vi "Main.vi"(11 "Module Admin":refnum<class "Delacor_lib_QMH_Module Admin.lvclass">) -> ()   [LabVIEW 2020, in "Config.lvlib"]
doc: "This template is based off of the Queued Message Handler design pattern and the Queued Message Handler project template that ships with LabVIEW.\n\nThe main difference is that the queue is private to this module and communication between modules is performed via Broadcast and Request events.\n\nRequest events are wrapped in public API methods and are handled in the Event Handling Loop (EHL) of this VI. Any module can register for Broadcast events sent by this module. The EHL generates messages based on user interface actions.\n\nThe Message Handling Loop (MHL) processes messages generated by the EHL, or by other messages. The messages are string values, so new messages can be added easily to the Message Cases case structure in the MHL. Each message cluster can also provide an optional value for Message Data, which is a variant that can be converted to whatever message-specific data is required.\n_____\nBased on Delacor QMH Project Template 5.0.0.82."
uses:
  Config.lvlib
  <vilib>/Delacor/Delacor QMH/Libraries/Module Admin_class/Delacor_lib_QMH_Module Admin.lvclass
  Acquisition/SignalConfig--cluster.ctl
  Module Data--cluster.ctl
  Stop Argument--cluster.ctl
  <vilib>/Delacor/Delacor QMH/Libraries/Message Queue_class/Delacor_lib_QMH_Message Queue.lvclass/Delacor_lib_QMH_Message Queue.ctl
  <vilib>/Delacor/Delacor QMH/Libraries/Module Admin_class/Delacor_lib_QMH_Module Admin.lvclass/Delacor_lib_QMH_Module Admin.ctl
  Save Config Argument--cluster.ctl
  Cancel config Argument--cluster.ctl
  Load Config Argument--cluster.ctl
  Load Config (Reply Payload)--cluster.ctl
  Config Loaded from DB Argument--cluster.ctl
  <vilib>/Utility/miscctls.llb/LVPointTypeDef.ctl
  <vilib>/Delacor/Delacor QMH/Libraries/Message Queue_class/Delacor_lib_QMH_Enqueue Message (Single).vi
  <vilib>/Delacor/Delacor QMH/Libraries/Module Admin_class/Delacor_lib_QMH_Get External Launch.vi
  <vilib>/Utility/error.llb/Error Cluster From Error Code.vi
  <vilib>/ErrorRing/Error Ring.xnode
  <vilib>/Delacor/Delacor QMH/Libraries/Message Queue_class/Delacor_lib_QMH_Message Queue.lvclass
  DataBase/DataBase.lvlib
panel:
  in  "SignalConfig":T1={"VPP"=0, "Frecuency"=50.0, "Offset"=0.0, "signal type"=enum."Sine Wave"}
  in  "Save":bool
  in  "Cancel":bool
  out "error out":errorcluster
  out "Status":string
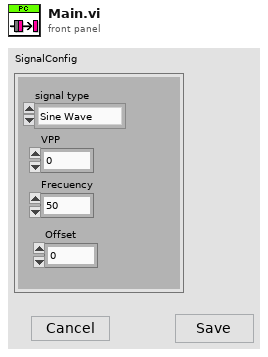
[diagram p1: front panel]
types:
  T1 = typedef "SignalConfig--cluster.ctl" = cluster{"VPP":i32, "Frecuency":dbl, "Offset":dbl, "signal type":enum16{"Sine Wave", "Triangle Wave", "Square Wave", "Sawtooth Wave"}}
  T2 = typedef "Config.lvlib/Request Events--cluster.ctl" = cluster{"Stop Module":refnum<user-event>, "Show Panel":refnum<user-event>, "Hide Panel":refnum<user-event>, "Get Module Execution Status":refnum<user-event>, "Show Diagram":refnum<user-event>, "Save Config":refnum<user-event>, "Cancel config":refnum<user-event>, "Load Config":refnum<user-event>, "Config Loaded from DB":refnum<user-event>}
  T3 = typedef "Config.lvlib/Module Data--cluster.ctl" = cluster{"Status":string, "SignalConfig":T1}
  T4 = enum32{"invalid lock state", "Not Locked", "Locked (No Password)", "Password-protected"}
  T5 = typedef "Config.lvlib/Stop Argument--cluster.ctl" = cluster{"Origin":string, "Exit via Stop Module Req?":bool, "Wait for Module to stop?":bool}
  T6 = typedef "Config.lvlib/Save Config Argument--cluster.ctl" = cluster{"Save":bool}
  T7 = typedef "Config.lvlib/Cancel config Argument--cluster.ctl" = cluster{"Cancel Button":bool}
  T8 = typedef "Config.lvlib/Load Config Argument--cluster.ctl" = cluster{"ID":dbl, "Wait Notifier":refnum<notifier>, "wait for reply":bool}
  T9 = typedef "Config.lvlib/Config Loaded from DB Argument--cluster.ctl" = cluster{"SignalConfig":T1}
  T10 = typedef "LVPointTypeDef.ctl" = cluster{"Horizontal":i16, "Vertical":i16}
  T11 = enum32{"Invalid", "Standard", "Closed", "Hidden", "Minimized", "Maximized"}
  T12 = typedef "Config.lvlib/Load Config (Reply Payload)--cluster.ctl" = cluster{"Config":bool, "Load Config_error":errorcluster}
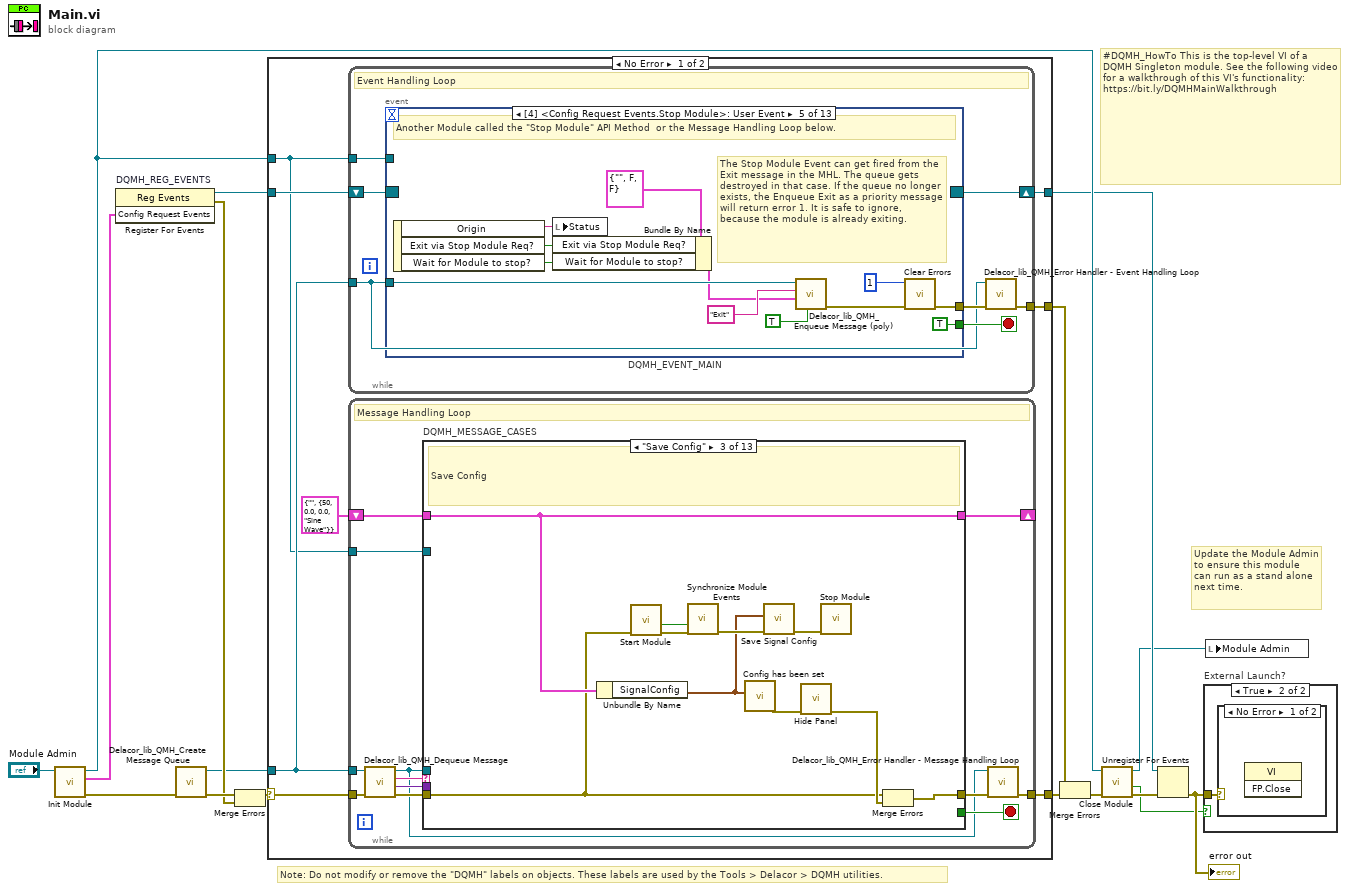
[diagram p0: block diagram]
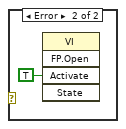
[diagram p3: hidden frame]
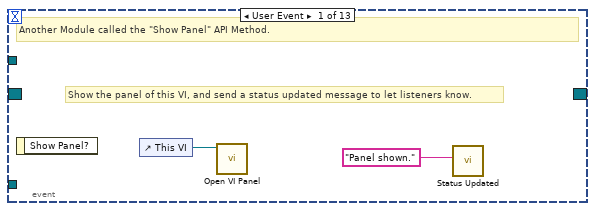
[diagram p4: hidden frame]
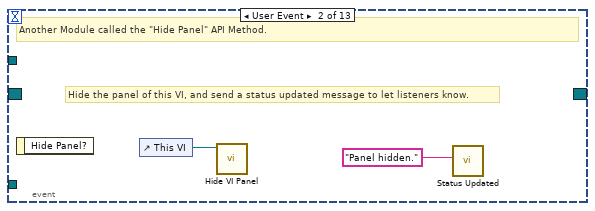
[diagram p5: hidden frame]
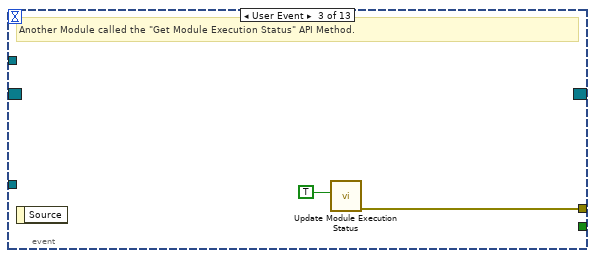
[diagram p6: hidden frame]
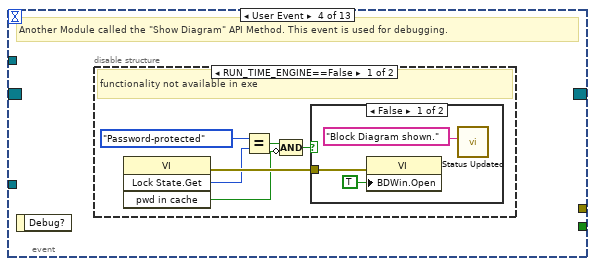
[diagram p7: hidden frame]
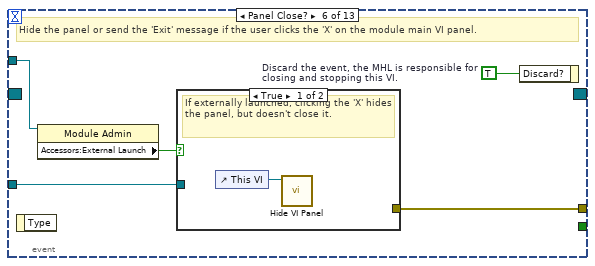
[diagram p10: hidden frame]
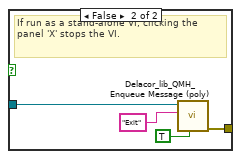
[diagram p11: hidden frame]
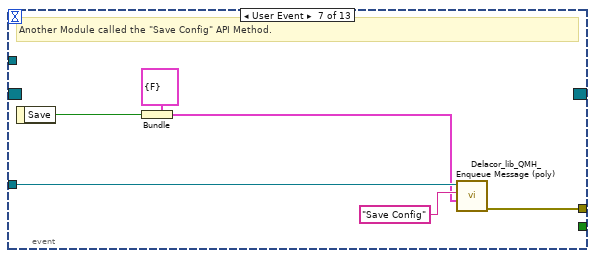
[diagram p12: hidden frame]
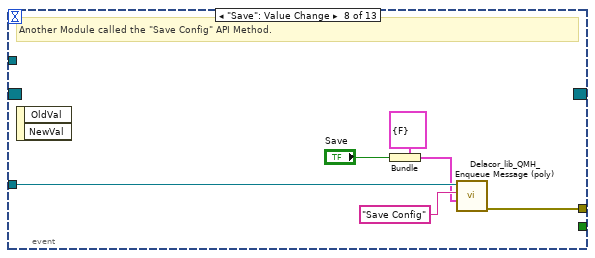
[diagram p13: hidden frame]
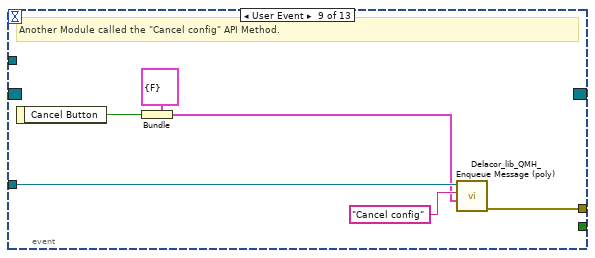
[diagram p14: hidden frame]
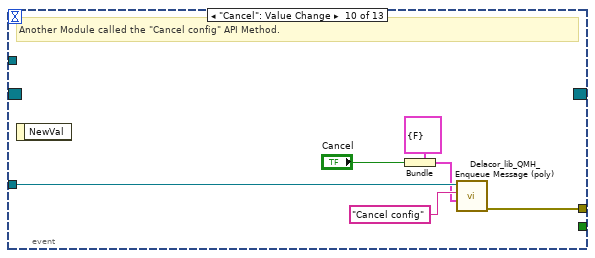
[diagram p15: hidden frame]
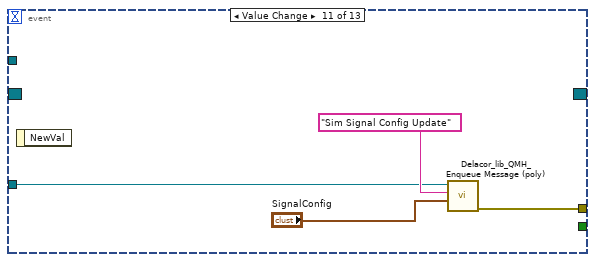
[diagram p16: hidden frame]
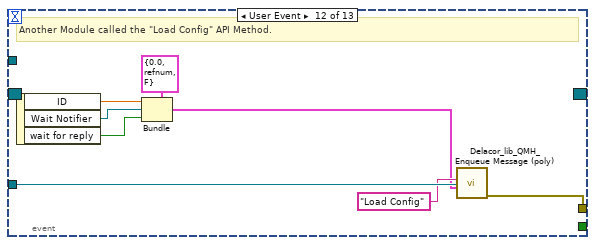
[diagram p17: hidden frame]
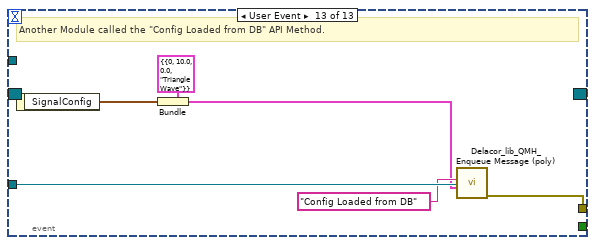
[diagram p18: hidden frame]
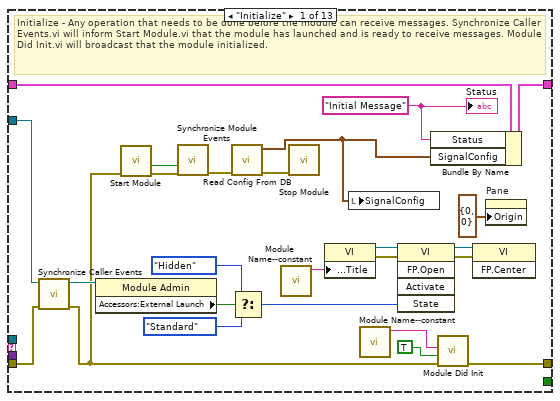
[diagram p19: hidden frame]
diagram:
  # "#DQMH_HowTo This is the top-level VI of a DQMH Singleton module. See the following video for a walkthrough of this VI's functionality: https://bit.ly/DQMHMainWalkthrough"
  # "Note: Do not modify or remove the \"DQMH\" labels on objects. These labels are used by the Tools > Delacor > DQMH utilities."
  # "Update the Module Admin to ensure this module can run as a stand alone next time."
  n1 = call "Init Module.vi"("Singleton Module Admin in"="Module Admin") -> ("error out"=w16:errorcluster, "Config Request Events"=w5:T2, "Singleton Module Admin out"=w8:refnum<class "Delacor_lib_QMH_Module Admin.lvclass">)  [unwired: 8 in]
  n2 = register-events "DQMH_REG_EVENTS"(w5) -> (reference out=w6:refnum<event-registration>, error out=w9:errorcluster)  [unwired: 2 in]
  n3 = call <vilib>:"Delacor_lib_QMH_Create Message Queue.vi"("error in"=w16) -> ("error out"=w11:errorcluster, "Message Queue"=w4:refnum<class "Delacor_lib_QMH_Message Queue.lvclass">)  [unwired: 9 in]
  n4 = Merge Errors(w11, w9) -> (w10:errorcluster)
  n5 = case shown="No Error" w10 {
    selector: w10 -> [w23 w263]
    tunnel: [w25 w262] -> w17
    tunnel: [w22 w268] -> w7
    tunnel: w6 -> [w20 w268]
    tunnel: w4 -> [w19 w261]
    tunnel: [w24 _] -> w14
    tunnel: w8 -> [w18 w264]
    frame No Error {
      n6 = while {
        tunnel: w19 -> [w26]
        shift-right: [w29] -> w22
        shift-left: w20 -> [w30]
        tunnel: [w31] -> w24
        tunnel: w18 -> [w27]
        stop <- w28 stop-if-true
        # "Event Handling Loop"
        n7 = event "DQMH_EVENT_MAIN" shown="[4] <Config Request Events.Stop Module>: User Event" {
          selector: w30 -> [_ _ _ _ _ _ _ _ _ _ _ _ _]
          dyn-events: [_ _ _ _ _ _ _ _ _ _ _ _ _] -> w29
          timeout: _ -> [_ _ _ _ _ _ _ _ _ _ _ _ _]
          tunnel: [_ _ _ _ TRUE ("Discard?") _ _ _ _ _ _ _ _] -> w28
          tunnel: w26 -> [_ _ _ _ w55 w62 w75 w81 w87 w93 w94 w105 w111]
          tunnel: [_ _ w38 _ w58 w64 w70 w77 w82 w89 w97 w98 w107] -> w32
          tunnel: w27 -> [_ _ _ _ _ w61 _ _ _ _ _ _ _]
          event User Event {
            # "Show the panel of this VI, and send a status updated message to let listeners know."
            # "Another Module called the \"Show Panel\" API Method."
            n8 = event-data() -> ()  [unwired: 1 in, 1 out]
            n9 = control-ref of="This VI"() -> (w34:refnum<vi>)
            n10 = call "Open VI Panel.vi"("VI"=w34) -> ()  [unwired: 10 in, 1 out]
            n11 = call "Status Updated.vi"("Status"="Panel shown." ("format string")) -> ()  [unwired: 10 in, 1 out]
          }
          event User Event {
            # "Hide the panel of this VI, and send a status updated message to let listeners know."
            # "Another Module called the \"Hide Panel\" API Method."
            n12 = event-data() -> ()  [unwired: 1 in, 1 out]
            n13 = control-ref of="This VI"() -> (w36:refnum<vi>)
            n14 = call "Hide VI Panel.vi"("VI"=w36) -> ()  [unwired: 10 in, 1 out]
            n15 = call "Status Updated.vi"("Status"="Panel hidden." ("format string")) -> ()  [unwired: 10 in, 1 out]
          }
          event User Event {
            # "Another Module called the \"Get Module Execution Status\" API Method."
            n16 = event-data() -> ()  [unwired: 1 in, 1 out]
            n17 = call "Update Module Execution Status.vi"("Running?"=TRUE) -> ("error out"=w38:errorcluster)  [unwired: 10 in]
          }
          event User Event {
            # "Another Module called the \"Show Diagram\" API Method. This event is used for debugging."
            n18 = event-data() -> ()  [unwired: 1 in, 1 out]
            n19 = disable-structure shown="RUN_TIME_ENGINE==False" {
              frame condition #0 (active) {
                # "functionality not available in exe"
                n20 = invoke class="VI" method="Lock State.Get"() -> (error out=w44:errorcluster, "Get Lock State"=w43:T4, "pwd in cache"=w40:bool)  [unwired: 4 in, 1 out]
                n21 = Equal?(x=T4."Password-protected", y=w43) -> (x = y?=w41:bool)
                n22 = Compound Arithmetic op=AND(w41, invert w40) -> (w39:bool)
                n23 = case shown="False" w39 {
                  tunnel: w44 -> [w47 _]
                  frame False {
                    n24 = property class="VI"(error in=w47, "BDWin.Open"=TRUE ("Block Diagram Window:Open")) -> ()  [unwired: 1 in, 2 out]
                    n25 = call "Status Updated.vi"("Status"="Block Diagram shown." ("format string")) -> ()  [unwired: 10 in, 1 out]
                  }
                  frame True {
                    # "Password-protected VI, and the password is not in the cache. Do not show the diagram."
                  }
                }
              }
              frame condition #1 {
              }
            }
          }
          event User Event {
            # "The Stop Module Event can get fired from the Exit message in the MHL. The queue gets destroyed in that case. If the queue no longer exists, the Enqueue Exit as a priority message will return error 1. It is safe to ignore, because the module is already exiting."
            # "Another Module called the \"Stop Module\" API Method  or the Message Handling Loop below."
            n26 = event-data() -> ("Origin"=w54:string, "Exit via Stop Module Req?"=w50:bool, "Wait for Module to stop?"=w49:bool)  [unwired: 1 in]
            n27 = local write "Status"(w54) -> ()
            n28 = Bundle By Name(cluster=T5 {"Origin"="", "Exit via Stop Module Req?"=FALSE, "Wait for Module to stop?"=FALSE} ("Stop Argument"), "Exit via Stop Module Req?"=w50, "Wait for Module to stop?"=w49) -> (w48:T5)
            n29 = call-poly <vilib>:"Delacor_lib_QMH_Enqueue Message (poly).vi"("Priority Message? (F)"=TRUE, "Message Data"=w48, "Message"="Exit", "Message Queue in"=w55) -> ("error out"=w59:errorcluster)  [unwired: 6 in, 1 out]
            n30 = call <vilib>:"Clear Errors.vi"("error in (no error)"=w59, "specific error code to clear (0: all)"=1) -> ("error out"=w58:errorcluster)  [unwired: 4 in, 1 out]
          }
          event Panel Close? {
            w63 = TRUE  # Discard the event, the MHL is responsible for closing and stopping this VI.
            # "Hide the panel or send the 'Exit' message if the user clicks the 'X' on the module main VI panel."
            n31 = event-data() -> ()  [unwired: 1 in, 1 out]
            n32 = property class="Module Admin"(reference=w61) -> ("Accessors:External Launch"=w60:bool)  [unwired: 1 in, 2 out]
            n33 = case shown="True" w60 {
              tunnel: w62 -> [_ w68]
              tunnel: [_ w69] -> w64
              frame True {
                # "If externally launched, clicking the 'X' hides the panel, but doesn't close it."
                n34 = control-ref of="This VI"() -> (w65:refnum<vi>)
                n35 = call "Hide VI Panel.vi"("VI"=w65) -> ()  [unwired: 10 in, 1 out]
              }
              frame False {
                # "If run as a stand-alone VI, clicking the panel 'X' stops the VI."
                n36 = call-poly <vilib>:"Delacor_lib_QMH_Enqueue Message (poly).vi"("Priority Message? (F)"=TRUE, "Message"="Exit", "Message Queue in"=w68) -> ("error out"=w69:errorcluster)  [unwired: 7 in, 1 out]
              }
            }
            n37 = event-data("Discard?"=w63) -> ()  [unwired: 1 in, 1 out]
          }
          event User Event {
            # "Another Module called the \"Save Config\" API Method."
            n38 = event-data() -> ("Save"=w71:bool)  [unwired: 1 in]
            n39 = Bundle(cluster=T6 {"Save"=FALSE} ("Save Config Argument"), "Save"=w71) -> (w72:T6)
            n40 = call-poly <vilib>:"Delacor_lib_QMH_Enqueue Message (poly).vi"("Message Data"=w72, "Message"="Save Config", "Message Queue in"=w75) -> ("error out"=w70:errorcluster)  [unwired: 7 in, 1 out]
          }
          event "Save": Value Change {
            # "Another Module called the \"Save Config\" API Method."
            n41 = event-data() -> ()  [unwired: 1 in, 2 out]
            n42 = Bundle(cluster=T6 {"Save"=FALSE} ("Save Config Argument"), "Save"="Save") -> (w78:T6)
            n43 = call-poly <vilib>:"Delacor_lib_QMH_Enqueue Message (poly).vi"("Message Data"=w78, "Message"="Save Config", "Message Queue in"=w81) -> ("error out"=w77:errorcluster)  [unwired: 7 in, 1 out]
          }
          event User Event {
            # "Another Module called the \"Cancel config\" API Method."
            n44 = event-data() -> ("Cancel Button"=w83:bool)  [unwired: 1 in]
            n45 = Bundle(cluster=T7 {"Cancel Button"=FALSE} ("Cancel config Argument"), "Cancel Button"=w83) -> (w84:T7)
            n46 = call-poly <vilib>:"Delacor_lib_QMH_Enqueue Message (poly).vi"("Message Data"=w84, "Message"="Cancel config", "Message Queue in"=w87) -> ("error out"=w82:errorcluster)  [unwired: 7 in, 1 out]
          }
          event "Cancel": Value Change {
            # "Another Module called the \"Cancel config\" API Method."
            n47 = event-data() -> ()  [unwired: 1 in, 1 out]
            n48 = Bundle(cluster=T7 {"Cancel Button"=FALSE} ("Cancel config Argument"), "Cancel Button"="Cancel") -> (w90:T7)
            n49 = call-poly <vilib>:"Delacor_lib_QMH_Enqueue Message (poly).vi"("Message Data"=w90, "Message"="Cancel config", "Message Queue in"=w93) -> ("error out"=w89:errorcluster)  [unwired: 7 in, 1 out]
          }
          event Value Change {
            n50 = event-data() -> ()  [unwired: 1 in, 1 out]
            n51 = call-poly <vilib>:"Delacor_lib_QMH_Enqueue Message (poly).vi"("Message Data"="SignalConfig", "Message"="Sim Signal Config Update", "Message Queue in"=w94) -> ("error out"=w97:errorcluster)  [unwired: 7 in, 1 out]
          }
          event User Event {
            # "Another Module called the \"Load Config\" API Method."
            n52 = event-data() -> ("ID"=w101:dbl, "Wait Notifier"=w100:refnum<notifier>, "wait for reply"=w99:bool)  [unwired: 1 in]
            n53 = Bundle(cluster=T8 {"ID"=0.0, "Wait Notifier"=refnum, "wait for reply"=FALSE} ("Load Config Argument"), "ID"=w101, "Wait Notifier"=w100, "wait for reply"=w99) -> (w102:T8)
            n54 = call-poly <vilib>:"Delacor_lib_QMH_Enqueue Message (poly).vi"("Message Data"=w102, "Message"="Load Config", "Message Queue in"=w105) -> ("error out"=w98:errorcluster)  [unwired: 7 in, 1 out]
          }
          event User Event {
            # "Another Module called the \"Config Loaded from DB\" API Method."
            n55 = event-data() -> ("SignalConfig"=w106:T1)  [unwired: 1 in]
            n56 = Bundle(cluster=T9 {"SignalConfig"={"VPP"=0, "Frecuency"=10.0, "Offset"=0.0, "signal type"=enum."Triangle Wave"}} ("Config Loaded from DB Argument"), "SignalConfig"=w106) -> (w108:T9)
            n57 = call-poly <vilib>:"Delacor_lib_QMH_Enqueue Message (poly).vi"("Message Data"=w108, "Message"="Config Loaded from DB", "Message Queue in"=w111) -> ("error out"=w107:errorcluster)  [unwired: 7 in, 1 out]
          }
        }
        n58 = call-dynamic "Delacor_lib_QMH_Error Handler - Event Handling Loop.vi"("error in"=w32, "Message Queue in"=w26) -> ("dup error in"=w31:errorcluster)  [unwired: 8 in, 1 out]
      }
      n59 = while {
        tunnel: w19 -> [w114]
        shift-right: [w118] -> _
        shift-left: T3 {"Status"="", "SignalConfig"={"VPP"=50, "Frecuency"=0.0, "Offset"=0.0, "signal type"=enum."Sine Wave"}} ("Data Cluster") -> [w119]
        tunnel: w23 -> [w122]
        tunnel: [w120] -> w25
        tunnel: w18 -> [w112]
        stop <- w117 stop-if-true
        # "Message Handling Loop"
        n60 = call-dynamic "Delacor_lib_QMH_Dequeue Message.vi"("error in"=w122, "Message Queue in"=w114) -> ("error out"=w121:errorcluster, "Message Data"=w115:variant, "Message"=w116:string, "Message Queue out"=w113:refnum<class "Delacor_lib_QMH_Message Queue.lvclass">)  [unwired: 6 in]
        n61 = case "DQMH_MESSAGE_CASES" shown="\"Save Config\"" w116 {
          selector: w116 -> [_ _ _ _ _ _ _ _ _ _ _ _ w248]
          tunnel: w113 -> [_ _ _ _ _ _ _ _ _ _ w218 w240 _]
          tunnel: w121 -> [w146 w150 w151 w167 w174 w186 w198 w201 w203 w208 w225 w246 w250]
          tunnel: [w145 w150 w158 w162 w172 w176 w191 w200 w203 w207 w221 w243 w251] -> w123
          tunnel: w119 -> [w136 w149 w160 w166 w173 w185 w197 w199 w202 w205 w220 w239 w249]
          tunnel: [w135 w149 w160 w166 w170 w185 w192 w199 w202 w205 w220 w239 w249] -> w118
          tunnel: [_ _ _ _ _ _ _ _ _ _ _ w238 _] -> w117
          tunnel: w115 -> [_ _ _ w164 w171 w183 w195 _ _ _ w219 w237 _]
          tunnel: w112 -> [w137 _ _ _ _ _ _ _ _ _ w217 w232 _]
          frame "Initialize" {
            w130 = "Initial Message" ("Initial Message")
            # "Initialize - Any operation that needs to be done before the module can receive messages. Synchronize Caller Events.vi will inform Start Module.vi that the module has launched and is ready to receive messages. Module Did Init.vi will broadcast that the module initialized."
            n62 = call "Synchronize Caller Events.vi"("error in (no error)"=w146, "Singleton Module Admin in"=w137) -> ("error out"=w124:errorcluster, "Singleton Module Admin out"=w132:refnum<class "Delacor_lib_QMH_Module Admin.lvclass">)  [unwired: 8 in]
            n63 = property class="Module Admin"(reference=w132) -> ("Accessors:External Launch"=w141:bool)  [unwired: 1 in, 2 out]
            n64 = call "Start Module.vi"("error in (no error)"=w124) -> ("error out"=w129:errorcluster, "Wait for Event Sync?"=w128:bool)  [unwired: 7 in, 2 out]
            n65 = call "Synchronize Module Events.vi"("error in (no error)"=w129, "Wait for Event Sync?"=w128) -> ("error out"=w127:errorcluster)  [unwired: 9 in]
            n66 = call "Read Config From DB.vi"("error in"=w127) -> ("error out"=w126:errorcluster, "SignalConfig"=w125:T1)  [unwired: 8 in, 1 out]
            n67 = Select(t=T11."Hidden" ("State"), s=w141, f=T11."Standard" ("State")) -> (s? t:f=w138:T11)
            n68 = call "Module Name--constant.vi"() -> ("Module Name"=w144:string)  [unwired: 11 in]
            n69 = call "Stop Module.vi"("error in (no error)"=w126) -> ()  [unwired: 10 in, 1 out]
            n70 = property class="VI"("Front Panel.Title"=w144) -> (reference out=w143:refnum<vi>, error out=w148:errorcluster)  [unwired: 2 in]
            n71 = local write "SignalConfig"(w125) -> ()
            n72 = call "Module Name--constant.vi"() -> ("Module Name"=w133:string)  [unwired: 11 in]
            n73 = invoke class="VI" method="FP.Open"(reference=w143, error in=w148, "State"=w138) -> (reference out=w142:refnum<vi>, error out=w147:errorcluster)  [unwired: 2 in, 3 out]
            n74 = Bundle By Name(cluster=w136, "Status"=w130, "SignalConfig"=w125) -> (w135:T3)
            n75 = call "Module Did Init.vi"("error in (no error)"=w124, "Initialized?"=TRUE, "Origin"=w133) -> ("error out"=w145:errorcluster)  [unwired: 8 in]
            n76 = invoke class="VI" method="FP.Center"(reference=w142, error in=w147) -> ()  [unwired: 1 in, 3 out]
            n77 = property on="Pane" class="Pane"("Origin"=T10 {"Horizontal"=0, "Vertical"=0}) -> ()  [unwired: 2 in, 2 out]
            "Status" <- w130
          }
          frame "--- Module Specific ---" {
            # "Separator -- The following cases handle messages specific to this Module."
          }
          frame "Save Config" {
            # "Save Config"
            n78 = Unbundle By Name(w160) -> ("SignalConfig"=w152:T1)
            n79 = call "Start Module.vi"("error in (no error)"=w151) -> ("error out"=w156:errorcluster, "Wait for Event Sync?"=w155:bool)  [unwired: 7 in, 2 out]
            n80 = call "Synchronize Module Events.vi"("error in (no error)"=w156, "Wait for Event Sync?"=w155) -> ("error out"=w154:errorcluster)  [unwired: 9 in]
            n81 = call "Config has been set.vi"("SignalConfig"=w152) -> ("error out"=w159:errorcluster)  [unwired: 10 in]
            n82 = call "Save Signal Config.vi"("error in"=w154, "SignalConfig"=w152) -> ("error out"=w153:errorcluster)  [unwired: 9 in]
            n83 = call "Hide Panel.vi"("error in (no error)"=w159) -> ("error out"=w157:errorcluster)  [unwired: 10 in]
            n84 = call "Stop Module.vi"("error in (no error)"=w153) -> ()  [unwired: 10 in, 1 out]
            n85 = Merge Errors(w151, w157) -> (w158:errorcluster)
          }
          frame "Cancel config" {
            # "Cancel config"
            n86 = Variant To Data(error in=w167, type=T7 {"Cancel Button"=FALSE} ("Cancel config Argument"), Variant=w164) -> (error out=w165:errorcluster)  [unwired: 1 out]
            n87 = call "Hide Panel.vi"() -> ("error out"=w161:errorcluster)  [unwired: 11 in]
            n88 = Merge Errors(w161, w165) -> (w162:errorcluster)
          }
          frame "Sim Signal Config Update" {
            n89 = Variant To Data(error in=w174, type=T1 {"VPP"=0, "Frecuency"=50.0, "Offset"=0.0, "signal type"=enum."Sine Wave"} ("SignalConfig"), Variant=w171) -> (data=w169:T1, error out=w172:errorcluster)
            n90 = Bundle By Name(cluster=w173, "SignalConfig"=w169) -> (w170:T3)
          }
          frame "Load Config" {
            # "Load config"
            n91 = Variant To Data(error in=w186, type=T8 {"ID"=0.0, "Wait Notifier"=refnum, "wait for reply"=FALSE} ("Load Config Argument"), Variant=w183) -> (data=w181:T8, error out=w184:errorcluster)
            n92 = Unbundle By Name(w181) -> ("Wait Notifier"=w180:refnum<notifier>, "wait for reply"=w179:bool)  [unwired: 1 out]
            n93 = Merge Errors(w184) -> (w176:errorcluster)
            n94 = Bundle By Name(cluster=T12 {"Config"=FALSE, "Load Config_error"={"status"=FALSE, "code"=0, "source"=""}} ("Load Config (Reply Payload)"), "Config"=TRUE) -> (w178:T12)
            n95 = case shown="True" w179 {
              tunnel: w180 -> [_ w188]
              tunnel: w178 -> [_ w187]
              frame False {
              }
              frame True {
                n96 = Send Notification(notification=w187, notifier=w188) -> ()  [unwired: 1 in, 2 out]
              }
            }
          }
          frame "Config Loaded from DB" {
            # "Config Loaded froma Data Base"
            n97 = Variant To Data(error in=w198, type=T9 {"SignalConfig"={"VPP"=0, "Frecuency"=10.0, "Offset"=0.0, "signal type"=enum."Triangle Wave"}} ("Config Loaded from DB Argument"), Variant=w195) -> (data=w193:T9, error out=w196:errorcluster)
            n98 = Unbundle By Name(w193) -> ("SignalConfig"=w189:T1)
            n99 = Bundle By Name(cluster=w197, "SignalConfig"=w189) -> (w192:T3)
            n100 = local write "SignalConfig"(w189) -> ()
            n101 = call "Config has been set.vi"("SignalConfig"=w189) -> ("error out"=w190:errorcluster)  [unwired: 10 in]
            n102 = Merge Errors(w196, w190) -> (w191:errorcluster)
          }
          frame "---Copy This Frame---" {
            # "Duplicate this frame when creating new messages.  Change this comment in the duplicated frame to describe this message."
            n103 = Merge Errors(w201) -> (w200:errorcluster)
          }
          frame "--- Exit and Error Handling---" {
            # "Separator - The following cases handle errors and exit messages."
          }
          frame "Simulate MHL Error" {
            # "#DQMH_HowTo The 'Simulate MHL Error' button  illustrates how the MHL handles errors. This event is instructional in nature and can be removed."
            # "Simulate an error occurring at the MHL"
            n104 = call "Module Name--constant.vi"() -> ("Module Name"=w204:string)  [unwired: 11 in]
            n105 = xnode "Error Ring"("parameter 0"=w204) -> ("error out"=w206:errorcluster)
            n106 = Merge Errors(w208, w206) -> (w207:errorcluster)
          }
          frame "Error" {
            # "Error - Check the error message data and respond accordingly. This message is sent by the \"Error Handler\" VIs at the end of each loop in this application."
            n107 = property class="Module Admin"(reference=w217) -> ("Accessors:External Launch"=w216:bool)  [unwired: 1 in, 2 out]
            n108 = Variant To Data(error in=w225, type=errorcluster {"status"=FALSE, "code"=0, "source"=""} ("error constant"), Variant=w219) -> (data=w226:errorcluster, error out=w223:errorcluster)
            n109 = call "Error Reported.vi"("Error"=w226) -> ()  [unwired: 10 in, 1 out]
            n110 = case shown="False" w216 {
              tunnel: [w231 _] -> w222
              tunnel: w218 -> [w229 _]
              tunnel: w226 -> [w230 _]
              frame False {
                # "If the module is running standalone, then pop up an error dialog and call the \"Exit\" message."
                n111 = call <vilib>:"Simple Error Handler.vi"("error in (no error)"=w230) -> ()  [unwired: 4 in, 5 out]
                n112 = call-poly <vilib>:"Delacor_lib_QMH_Enqueue Message (poly).vi"("Priority Message? (F)"=TRUE, "Message"="Exit", "Message Queue in"=w229) -> ("error out"=w231:errorcluster)  [unwired: 7 in, 1 out]
              }
              frame True {
                # "If the module was launched externally, calling the Error Reported broadcast VI is the only action performed by the \"Error\" message. The module's caller can then process the error appropriately."
              }
            }
            n113 = Merge Errors(w223, w222) -> (w221:errorcluster)
            n114 = local write "error out"(w221) -> ()
          }
          frame "Exit" {
            w236 = 91  # 91: not all Exit messages will have an argument
            w238 = TRUE  # Stop the VI
            # "Release the message queue reference"
            # "#CodeNeeded - Add any required cleanup code here"
            # "Exit - Exit the application."
            n115 = Variant To Data(error in=w246, type=T5 {"Origin"="", "Exit via Stop Module Req?"=FALSE, "Wait for Module to stop?"=FALSE} ("Stop Argument"), Variant=w237) -> (data=w234:T5, error out=w242:errorcluster)
            n116 = call <vilib>:"Clear Errors.vi"("error in (no error)"=w242, "specific error code to clear (0: all)"=w236) -> ("error out"=w245:errorcluster)  [unwired: 4 in, 1 out]
            n117 = control-ref of="This VI"() -> (w233:refnum<vi>)
            n118 = call-dynamic "Delacor_lib_QMH_Release Message Queue.vi"("error in"=w245, "Message Queue"=w240) -> ("error out"=w244:errorcluster)  [unwired: 9 in]
            n119 = call "Handle Exit.vi"("Stop Argument"=w234, "Admin in"=w232, "VI reference"=w233) -> ("error out"=w241:errorcluster)  [unwired: 7 in, 1 out]
            n120 = Merge Errors(w244, w241) -> (w243:errorcluster)
          }
          frame Default {
            # "'Default' case only runs if there is a message that isn't defined in any of the other cases.  Output a programming error."
            n121 = call "Module Name--constant.vi"() -> ("Module Name"=w247:string)  [unwired: 11 in]
            n122 = xnode "Error Ring"("parameter 0"=w248, "parameter 1"=w247) -> ("error out"=w252:errorcluster)
            n123 = Merge Errors(w250, w252) -> (w251:errorcluster)
          }
        }
        n124 = call-dynamic "Delacor_lib_QMH_Error Handler - Message Handling Loop.vi"("error in"=w123, "Message Queue in"=w113) -> ("dup error in"=w120:errorcluster)  [unwired: 8 in, 1 out]
      }
    }
    frame Error {
      # "Synchronize Caller Events.vi will inform Start Module.vi that the module has launched and will let the code calling Start Module.vi register for broadcasts and would permit the caller receive the broadcast that an error occurred at launch time."
      n125 = call-dynamic "Delacor_lib_QMH_Release Message Queue.vi"("error in"=w263, "Message Queue"=w261) -> ("error out"=w262:errorcluster)  [unwired: 9 in]
      n126 = call "Synchronize Caller Events.vi"("Singleton Module Admin in"=w264) -> ("error out"=w269:errorcluster)  [unwired: 9 in, 1 out]
      n127 = call "Module Name--constant.vi"() -> ("Module Name"=w267:string)  [unwired: 11 in]
      n128 = Format Into String(format string="An error occurred during initialization. %s is no longer running.", w267) -> (resulting string=w265:string)  [unwired: 2 in, 1 out]
      n129 = Merge Errors(w262, w269) -> (w270:errorcluster)
      n130 = call "Error Reported.vi"("Additional Information"=w265, "Error"=w270) -> ()  [unwired: 9 in, 1 out]
    }
  }
  n131 = Merge Errors(w14, w17) -> (w13:errorcluster)
  n132 = call "Close Module.vi"("error in (no error)"=w13, "Module Admin in"=w8) -> ("error out"=w15:errorcluster, "External Launch"=w1:bool, "Module Admin out"=w2:refnum<class "Delacor_lib_QMH_Module Admin.lvclass">)  [unwired: 7 in]
  n133 = Unregister For Events(event registration refnum=w7, error in=w15) -> (error out=w12:errorcluster)
  "error out" <- w12
  n134 = case "External Launch?" shown="True" w1 {
    tunnel: w12 -> [_ w271]
    frame False {
    }
    frame True {
      n135 = case shown="No Error" w271 {
        frame No Error {
          n136 = invoke class="VI" method="FP.Close"() -> ()  [unwired: 3 in, 3 out]
        }
        frame Error {
          n137 = invoke class="VI" method="FP.Open"("Activate"=TRUE ("Activate?")) -> ()  [unwired: 4 in, 5 out]
        }
      }
    }
  }
  n138 = local write "Module Admin"(w2) -> ()
